vi "data_que.vi"() -> (0 "error out":errorcluster, 3 "DATA_QUEUE":refnum<queue>)   [LabVIEW 2013]
uses:
  main_machine/type_defs/data_message.ctl
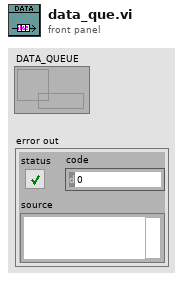
[diagram p1: front panel]
types:
  T1 = typedef "data_message.ctl" = enum16{"INITIALIZE", "UPDATE DATA", "THROW AWAY DATA", "ANALYZE DATA", "SAVE DATA", "SHUTDOWN"}
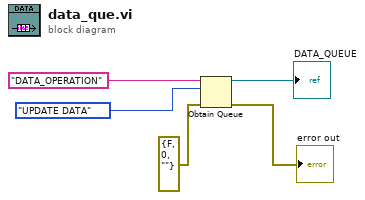
[diagram p0: block diagram]
diagram:
  n1 = Obtain Queue(name (unnamed)="DATA_OPERATION", element data type=data_message."UPDATE DATA", error in (no error)=errorcluster {"status"=FALSE, "code"=0, "source"=""}) -> (queue out=→"DATA_QUEUE":refnum<queue>, error out=→"error out":errorcluster)  [unwired: 2 in, 1 out]
